vi "Enqueue Multi Name.vi"(6 "Priority":T1, 8 "error in":errorcluster, 10 "States":string[](array[string]), 11 "QDMH in":refnum<class "QDMH.lvclass">) -> (0 "error out":errorcluster, 3 "QDMH out":refnum<class "QDMH.lvclass">)   [LabVIEW 2023, in "QDMH.lvlib" / "QDMH.lvclass"]
uses:
  QDMH.lvclass
  Custom Controls/Priority.ctl
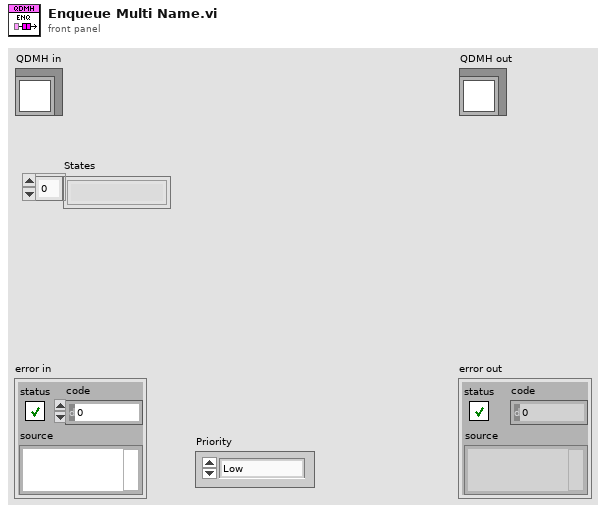
[diagram p1: front panel]
types:
  T1 = typedef "QDMH.lvlib/QDMH.lvclass/Priority.ctl" = enum16{"Low ", "High"}
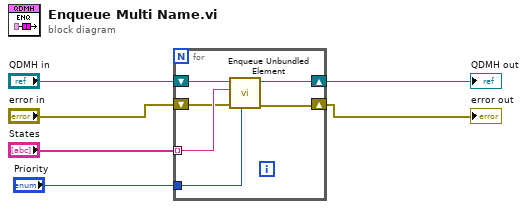
[diagram p0: block diagram]
diagram:
  n1 = for {
    shift-right: [w11] -> w3
    shift-left: "QDMH in" -> [w12]
    tunnel: "States" -> [w10] mode=indexing
    shift-right: [w9] -> w5
    shift-left: "error in" -> [w8]
    tunnel: "Priority" -> [w7]
    n2 = call "Enqueue Unbundled Element.vi"("Priority"=w7, "error in"=w8, "State"=w10, "QDMH in"=w12) -> ("error out"=w9:errorcluster, "QDMH out"=w11:refnum<class "QDMH.lvclass">)  [unwired: 6 in]
  }
  "error out" <- w5
  "QDMH out" <- w3
